vi "_PC_RTFunc_AccessD999.vi"(7 "Function":enum16{"WriteCmd", "ReadParam", "ReadResponse"}(ring), 8 "error in (no error)":errorcluster, 9 "Variant":variant, 11 "Cmd":string) -> (0 "error out":errorcluster, 2 "D999_Param":T1={"Enable"=FALSE, "AI"=[{"Label"="", "MultiValue"=1.0, "AddValue"=0.0}, {"Label"="", "MultiValue"=1.0, "AddValue"=0.0}, {"Label"="", "MultiValue"=1.0, "AddValue"=0.0}, {"Label"="", "MultiValue"=1.0, "AddValue"=0.0}, {"Label"="", "MultiValue"=1.0, "AddValue"=0.0}, {"Label"="", "MultiValue"=1.0, "AddValue"=0.0}, {"Label"="", "MultiValue"=1.0, "AddValue"=0.0}, {"Label"="", "MultiValue"=1.0, "AddValue"=0.0}, {"Label"="", "MultiValue"=1.0, "AddValue"=0.0}, {"Label"="", "MultiValue"=1.0, "AddValue"=0.0}, {"Label"="", "MultiValue"=1.0, "AddValue"=0.0}, {"Label"="", "MultiValue"=1.0, "AddValue"=0.0}], "AO"=[], "Switch"=[]})   [LabVIEW 2018]
uses:
  RT/PublicSubVI/Ctl/_ctl_RT_D999_Param.ctl
  RT/PublicSubVI/Ctl/_ctl_RT_D999_Command.ctl
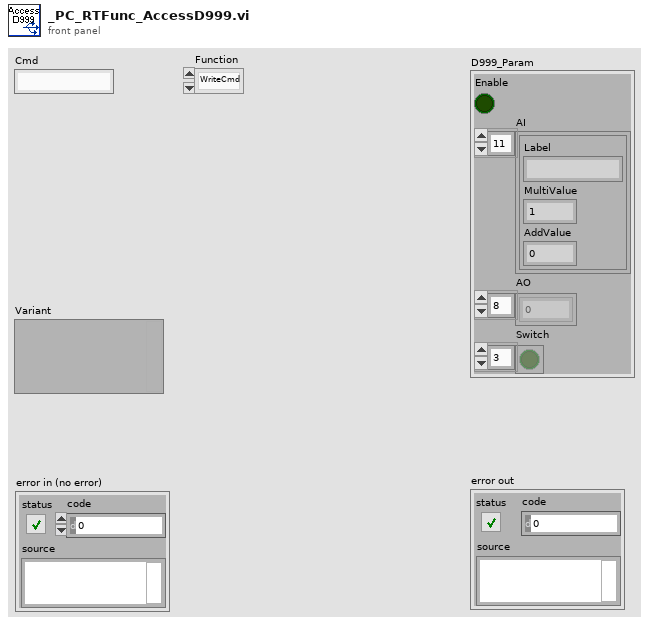
[diagram p1: front panel]
types:
  T1 = typedef "_ctl_RT_D999_Param.ctl" = cluster{"Enable":bool, "AI":cluster{"Label":string, "MultiValue":dbl, "AddValue":dbl}[], "AO":i16[], "Switch":bool[]}
  T2 = typedef "_ctl_RT_D999_Command.ctl" = cluster{"label":string, "value":variant}
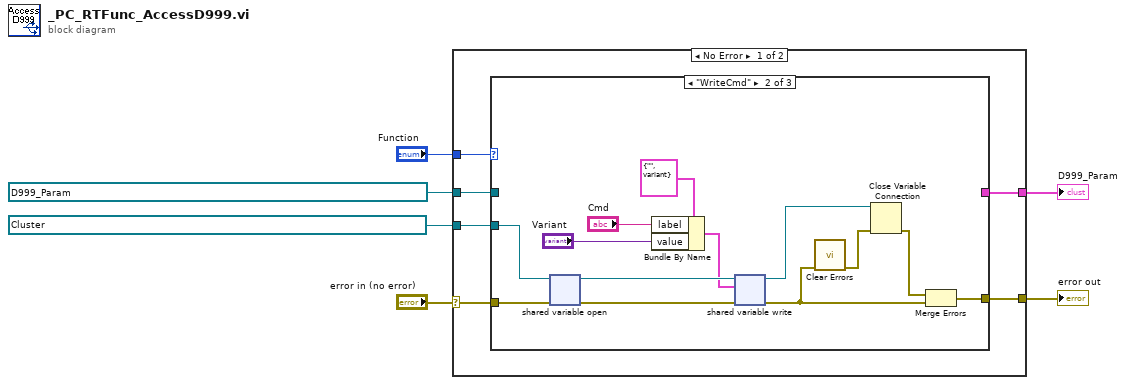
[diagram p0: block diagram]
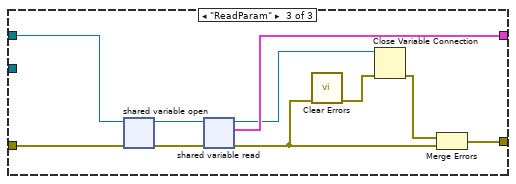
[diagram p3: hidden frame]
diagram:
  n1 = case shown="No Error" "error in (no error)" {
    selector: "error in (no error)" -> [w7 w37]
    tunnel: [w12 _] -> w6
    tunnel: [w8 w37] -> w5
    tunnel: refnum<k21> "ni.var.psp://NI-sbRIO/_RT_CtrlLoop_D999_Variables/D999_UserParam" ("shared variable refnum in") -> [w11 _]
    tunnel: refnum<k21> "ni.var.psp://NI-sbRIO/_RT_CtrlLoop_D999_Variables/D999_Command" ("shared variable refnum in") -> [w10 _]
    tunnel: "Function" -> [w9 _]
    frame No Error {
      n2 = case shown="\"WriteCmd\"" w9 {
        tunnel: [_ _ w32] -> w12
        tunnel: [w13 w15 w27] -> w8
        tunnel: w7 -> [w13 w24 w35]
        tunnel: w11 -> [_ _ w36]
        tunnel: w10 -> [_ w23 _]
        frame Default {
        }
        frame "WriteCmd" {
          n3 = shared-variable-open(w23, w24) -> (w22:refnum<k21>, w21:errorcluster)
          n4 = Bundle By Name(cluster=T2 {"label"="", "value"=variant} ("Cluster"), "label"="Cmd", "value"="Variant") -> (w20:T2)
          n5 = shared-variable-write(w22, w21, w20) -> (w19:refnum<k21>, w16:errorcluster)
          n6 = call <vilib>:"Clear Errors.vi"("error in (no error)"=w16) -> ("error out"=w18:errorcluster)  [unwired: 5 in, 1 out]
          n7 = Close Variable Connection(8:w18, 11:w19) -> (0:w17:errorcluster)
          n8 = Merge Errors(w17, w16) -> (w15:errorcluster)
        }
        frame "ReadParam" {
          n9 = shared-variable-open(w36, w35) -> (w34:refnum<k21>, w33:errorcluster)
          n10 = shared-variable-read(w34, w33) -> (w30:refnum<k21>, w28:errorcluster, w32:T1)
          n11 = call <vilib>:"Clear Errors.vi"("error in (no error)"=w28) -> ("error out"=w31:errorcluster)  [unwired: 5 in, 1 out]
          n12 = Close Variable Connection(8:w31, 11:w30) -> (0:w29:errorcluster)
          n13 = Merge Errors(w29, w28) -> (w27:errorcluster)
        }
      }
    }
    frame Error {
    }
  }
  "D999_Param" <- w6
  "error out" <- w5
